vi "uAssembler_Launch.vi"(0 "Path":path) -> ()   [LabVIEW 2021, in "uAssembler.lvlib" / "uAssembler.lvclass"]
doc: "To use this VI, use a \"call-by-reference\" node in the caller VI and pass in the lvclass filepath.\nThe caller shall not be statically linked to any classes. It is meant to be a lightweight splashscreen without any dependencies.\n\nWhere needed, use a special queue named 'splash' to report the progress in loading classes without creating a static dependency between the caller and the callee."
uses:
  uAssembler.lvclass
  Bin/uFramework.lvlibp/uTransport_uActor/uTransport_uActor.lvclass
  uAssembler.lvclass/uAssembler.ctl
  <vilib>/Utility/Data Type/NI_Data Type.lvlib
  Bin/uFramework.lvlibp/uActor/uActor.lvclass
  U:/Projects/uFramework/Src/uFramework_pack_uActor/uObserver/uObserver.lvclass
  U:/Projects/uFramework/Bin/uFramework.lvlibp/uActor/uActor.lvclass
  U:/Projects/uFramework/Bin/uFramework.lvlibp/uTransport/uTransport.lvclass
  U:/Projects/uFramework/Src/uFramework_pack_uActor/uAssembler/uAssembler.lvclass
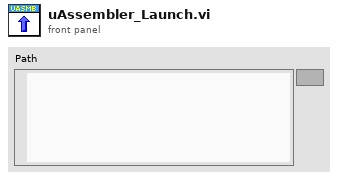
[diagram p1: front panel]
types:
  T1 = enum32{"Invalid", "Standard", "Closed", "Hidden", "Minimized", "Maximized"}
  T2 = typedef "Member VI Info.ctl" = cluster{"qualified name":string, "path":path, "access scope":enum32{"invalid scope", "public", "private", "protected", "community"}, "is dynamic dispatch":bool}
  T3 = enum32{"invalid app kind", "Development System", "Run Time System", "Student Edition", "Embedded LabVIEW", "Evaluation", "Custom"}
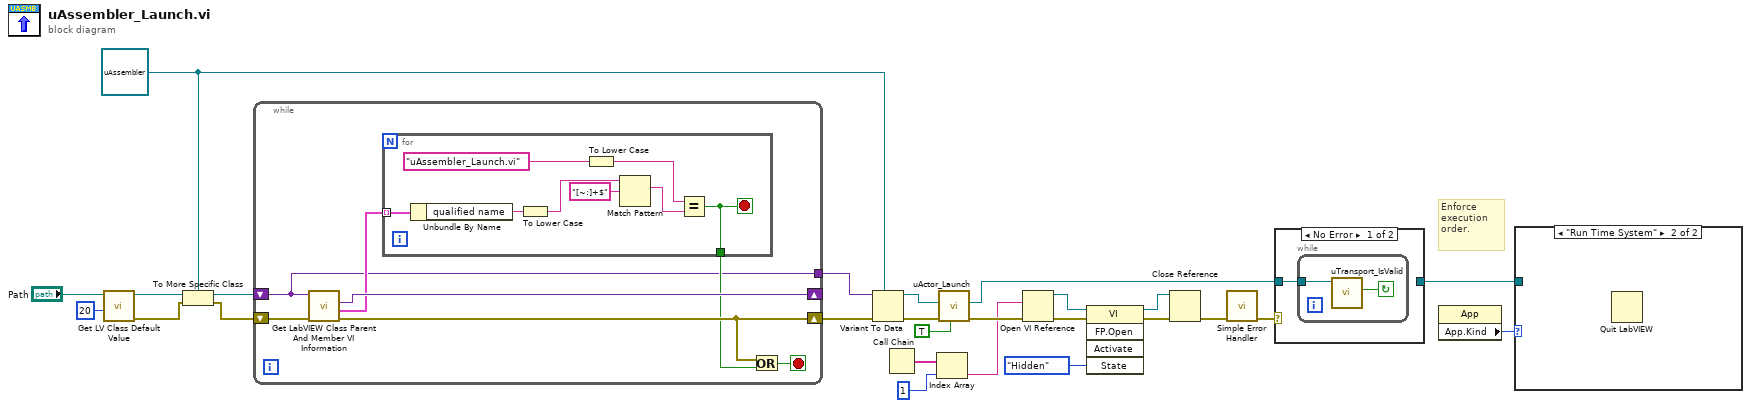
[diagram p0: block diagram]
diagram:
  w13 = refnum<class "uAssembler.lvclass"> refnum ("uAssembler.lvlib:uAssembler.lvclass")
  # "Enforce execution order."
  n1 = call <vilib>:"Get LV Class Default Value.vi"("options"=u32 20, "class path"="Path") -> ("error out"=w15:errorcluster, "object"=w19:refnum<class>)  [unwired: 8 in]
  n2 = To More Specific Class(target class=w13, reference=w19, error in=w15) -> (specific class reference=w16:refnum<class "uAssembler.lvclass">, error out=w14:errorcluster)
  n3 = while {
    shift-right: [w30] -> w25
    shift-left: w14 -> [w32]
    shift-right: [w33] -> _
    shift-left: w16 -> [w27]
    tunnel: [w27] -> w26
    stop <- w28 stop-if-true
    n4 = call <vilib>:"Get LabVIEW Class Parent And Member VI Information.vi"("error in (no error)"=w32, "variant"=w27) -> ("error out"=w30:errorcluster, "member VI info"=w31:T2[], "parent class"=w33:variant)  [unwired: 6 in, 1 out]
    n5 = for {
      tunnel: w31 -> [w36] mode=indexing
      tunnel: [w35] -> w29
      stop <- w35 stop-if-true
      n6 = Unbundle By Name(w36) -> ("qualified name"=w41:string)
      n7 = To Lower Case(string=w41) -> (all lower case string=w39:string)
      n8 = To Lower Case(string="uAssembler_Launch.vi" ("x")) -> (all lower case string=w34:string)
      n9 = Match Pattern(string=w39, regular expression="[~:]+$") -> (match substring=w38:string)  [unwired: 1 in, 3 out]
      n10 = Equal?(x=w34, y=w38) -> (x = y?=w35:bool)
    }
    n11 = Or(x=w30, y=w29) -> (x .or. y?=w28:bool)
  }
  n12 = Variant To Data(error in=w25, type=w13, Variant=w26) -> (data=w23:refnum<class "uAssembler.lvclass">, error out=w24:errorcluster)
  n13 = Call Chain() -> (call chain=w12:string[])
  n14 = Index Array(array=w12, index=1) -> (element=w7:string)
  n15 = call "uActor_Launch.vi"("Show FP (F)"=TRUE, "error in (no error)"=w24, "Actor to Launch"=w23) -> ("error out"=w9:errorcluster, "uTransport_uActor"=w21:refnum<class "uTransport_uActor.lvclass">)  [unwired: 6 in, 1 out]
  n16 = Open VI Reference(vi path=w7, error in (no error)=w9) -> (vi reference=w6:refnum<vi>, error out=w8:errorcluster)  [unwired: 4 in]
  n17 = invoke class="VI" method="FP.Open"(reference=w6, error in=w8, "State"=T1."Hidden") -> (reference out=w3:refnum<vi>, error out=w10:errorcluster)  [unwired: 2 in, 3 out]
  n18 = Close Reference(reference=w3, error in (no error)=w10) -> (error out=w4:errorcluster)
  n19 = call <vilib>:"Simple Error Handler.vi"("error in (no error)"=w4) -> ("error out"=w20:errorcluster)  [unwired: 4 in, 4 out]
  n20 = case shown="No Error" w20 {
    tunnel: w21 -> [w42 w45]
    tunnel: [_ w45] -> w1
    frame No Error {
      n21 = while {
        tunnel: w42 -> [w43]
        stop <- w44 continue-if-true
        n22 = call-dynamic "uTransport_IsValid.vi"("uTransport_uActor in"=w43) -> ("IsValid?"=w44:bool)  [unwired: 8 in, 2 out]
      }
    }
    frame Error {
    }
  }
  n23 = property class="App"() -> ("App.Kind"=w2:T3)  [unwired: 2 in, 2 out]
  n24 = case shown="\"Run Time System\"" w2 {
    tunnel: w1 -> [_ _]
    frame Default {
    }
    frame "Run Time System" {
      n25 = Quit LabVIEW() -> ()  [unwired: 1 in]
    }
  }
